vi "app - view -- guided sweep - V2.vi"() -> ()   [LabVIEW 2015]
uses:
  type - has been touched.ctl
  ctl -- name dispatcher -- action.ctl
  next chunk read-write PID -- action.ctl
  cursor action.ctl
  ctl -- name dispatcher.vi
  file -- 9w path.vi
  array -- find index - real.vi
  array -- interpolate -- i.vi
  tale of three indices.vi
  linear interpolation - real.vi
  line -- complex.vi
  Q -- check range -- i -- integer.vi
  Q -- check range -- i -- real.vi
  command stack.vi
  tale of three indices -- check state.vi
  Q - not nan -- integer.vi
  Q - not nan -- real.vi
  <vilib>/Utility/libraryn.llb/Check if File or Folder Exists.vi
  file -- read list of lines.vi
  parse -- find first line.vi
  parse -- get list of matches -- numbers.vi
  <vilib>/Utility/file.llb/Write To Spreadsheet File.vi
  <vilib>/Utility/file.llb/Write To Spreadsheet File (string).vi
  <vilib>/gmath/function.llb/Binomial Coefficient.vi
panel:
  in  "Tab Control 2":enum32{"main", "other"}(tab)
  out "Plot: Temp vs Time":cluster{dbl[], dbl[]}[](graph)=[{[0.0, 644.73684, 3070.17544, 4635.96491, 6278.50877], [60.0, 115.47619, 164.28571, 228.57143, 294.04762]}, {array[1000 elements], array[1000 elements]}]
  in  "sweep folder path":path=path "D:/Technique/RUS/LSCO/LSCO22_130814c_polished_Fenix/0_test"
  out "Plot: T slope":cluster{dbl[], dbl[]}[](graph)
  out "Plot:  dT  vs T":cluster{dbl[], dbl[]}[](graph)
  in  "divide T by":i32=1
  in  "time min":dbl(slide)=0.01167520658858774 min=-506096563.00000006 max=2129711151.0 step=0.010000000000000002 scale=0.01..1000.0 scale format="%#3_3f"
  in  "Time max":dbl(slide)=6895.4882445737985 min=-506096563.00000006 max=2129711151.0 step=0.010000000000000002 scale=0.01..10000.0 scale format="%#3_3f"
  in  "N":i32(slide)=438 min=-506096563 max=2129711151 step=1 scale=0.01..1000.0
  out "Plot: voltage":cluster{dbl[], dbl[]}[](graph)=[{[5.0, 30.0, 60.0, 100.0, 300.0], [0.1, 0.3, 0.5, 0.5, 1.5]}, {array[1000 elements], array[1000 elements]}]
  out "Plot: K/sweep vs T":cluster{dbl[], dbl[]}[](graph)
  out "Plot: (min)/sweep vs T":cluster{dbl[], dbl[]}[](graph)
  in  "Current time":timestamp=timestamp(3536522640.967544 s since 1904-01-01) format="%<%A, %b%d , %I:%M:%S%p>T"
  out "time at yellow cursor":timestamp=timestamp(3536726193.599123 s since 1904-01-01) format="%<%A, %b%d , %I:%M:%S%p>T"
  out "temperature":dbl
  in  "update bezier!":bool
  in  "update file on disk":bool
  in  "Tab Control":enum32{"fancy", "old"}(tab)
  out "new time":dbl[](array[numeric])=[0.0, 660.0877192982456, 3070.17544, 4635.96491, 6278.50877]
  out "new temperature":dbl[](array[numeric])=[60.0, 115.47619047619048, 164.28571, 228.57143, 294.04762]
  out "time":dbl[](array[numeric])=[0.0, 644.73684, 3070.17544, 4635.96491, 6278.50877]
  out "temperature":dbl[](array[numeric])=[60.0, 115.47619, 164.28571, 228.57143, 294.04762]
  in  "weights":dbl[](array[numeric])=[2.0, 5.0, 1.0, 1.0, 1.0]
  in  "weights changed":T1
  out "header":string[](array[string])=["# set temperature PID", "# Time ", "# set temperature", "# weight", "", "#cooling"]
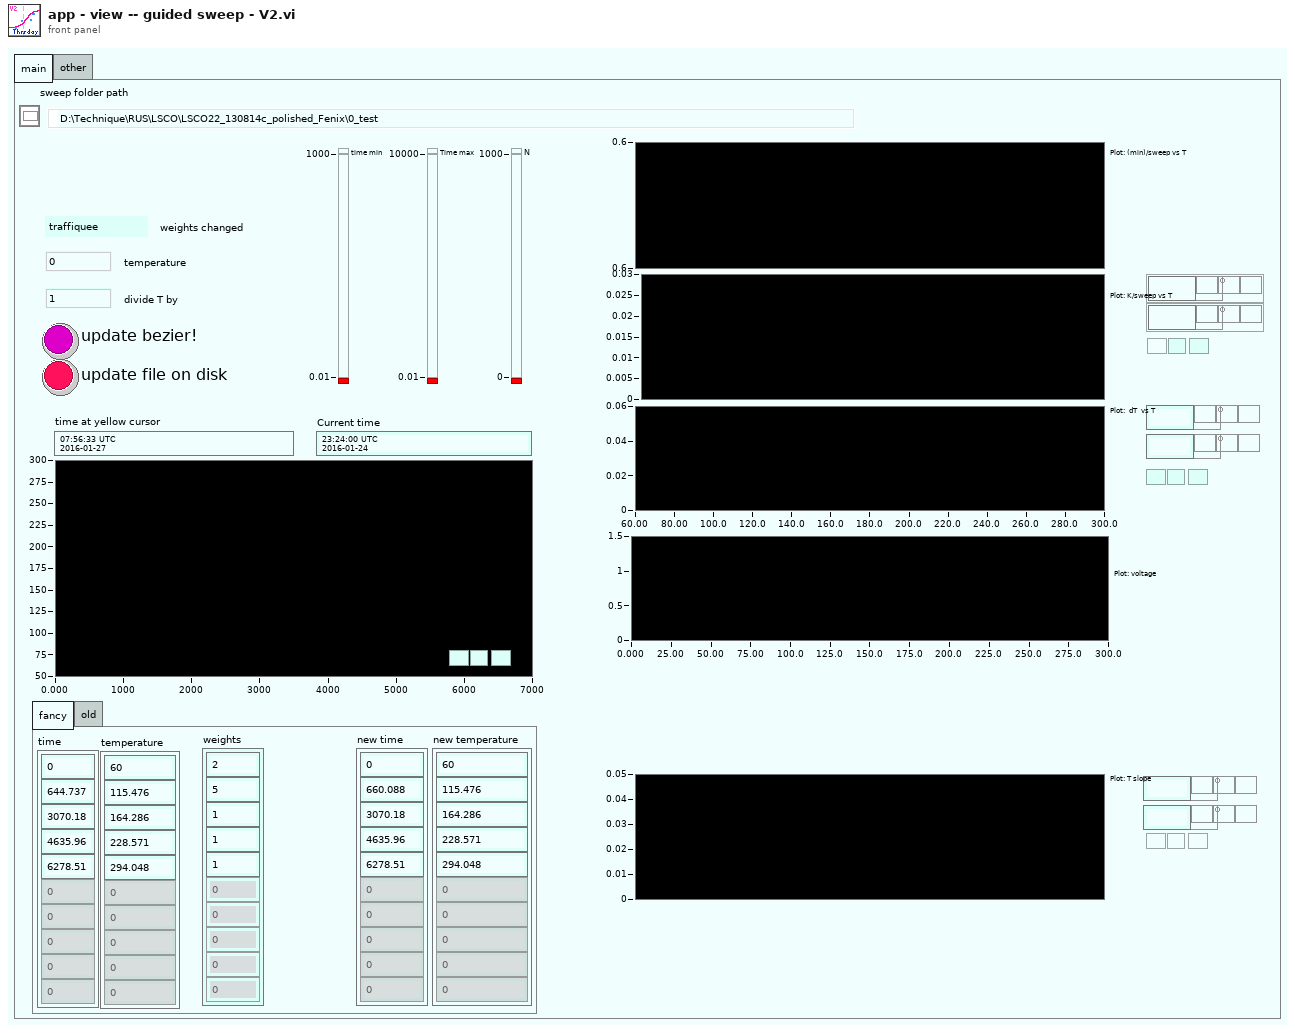
[diagram p1: front panel]
types:
  T1 = typedef "type - has been touched.ctl" = enum16{"traffiquee", "clean"}
  T2 = typedef "next chunk read-write PID -- action.ctl" = enum16{"read", "interpolate", "append col", "write", "write PID col", "append PID col", "interpolate - bezier"}
  T3 = typedef "ctl -- name dispatcher -- action.ctl" = enum16{"peak frequency", "peak frequency DUMP", "peak gamma DUMP", "peak gamma", "peak frequency TEST", "peak gamma TEST", "ultrasonic power", "time in gamma", "set temperature ", "set temperature timer", "peak default gamma", "last scan file", "peak freq gamma TEST", "peak NAMES", "errors", "P_I_D", "P", "I", "D", "power vs time", "power vs time TIMER", "void", "power log", "set temperature - SINE", "itc ltc log", "peak - time in gamma"}
  T4 = enum16{"normal", "alert", "fuzzy", "interesting", "boring", "colored"}
  T5 = typedef "cursor action.ctl" = enum16{"range", "read", "write", "check", "zoom out", "smart zoom out"}
  T6 = cluster{"temperatures":dbl[], "frequencies":dbl[]}
  T7 = cluster{"temperatures":dbl[], "frequencies":dbl[]}[]
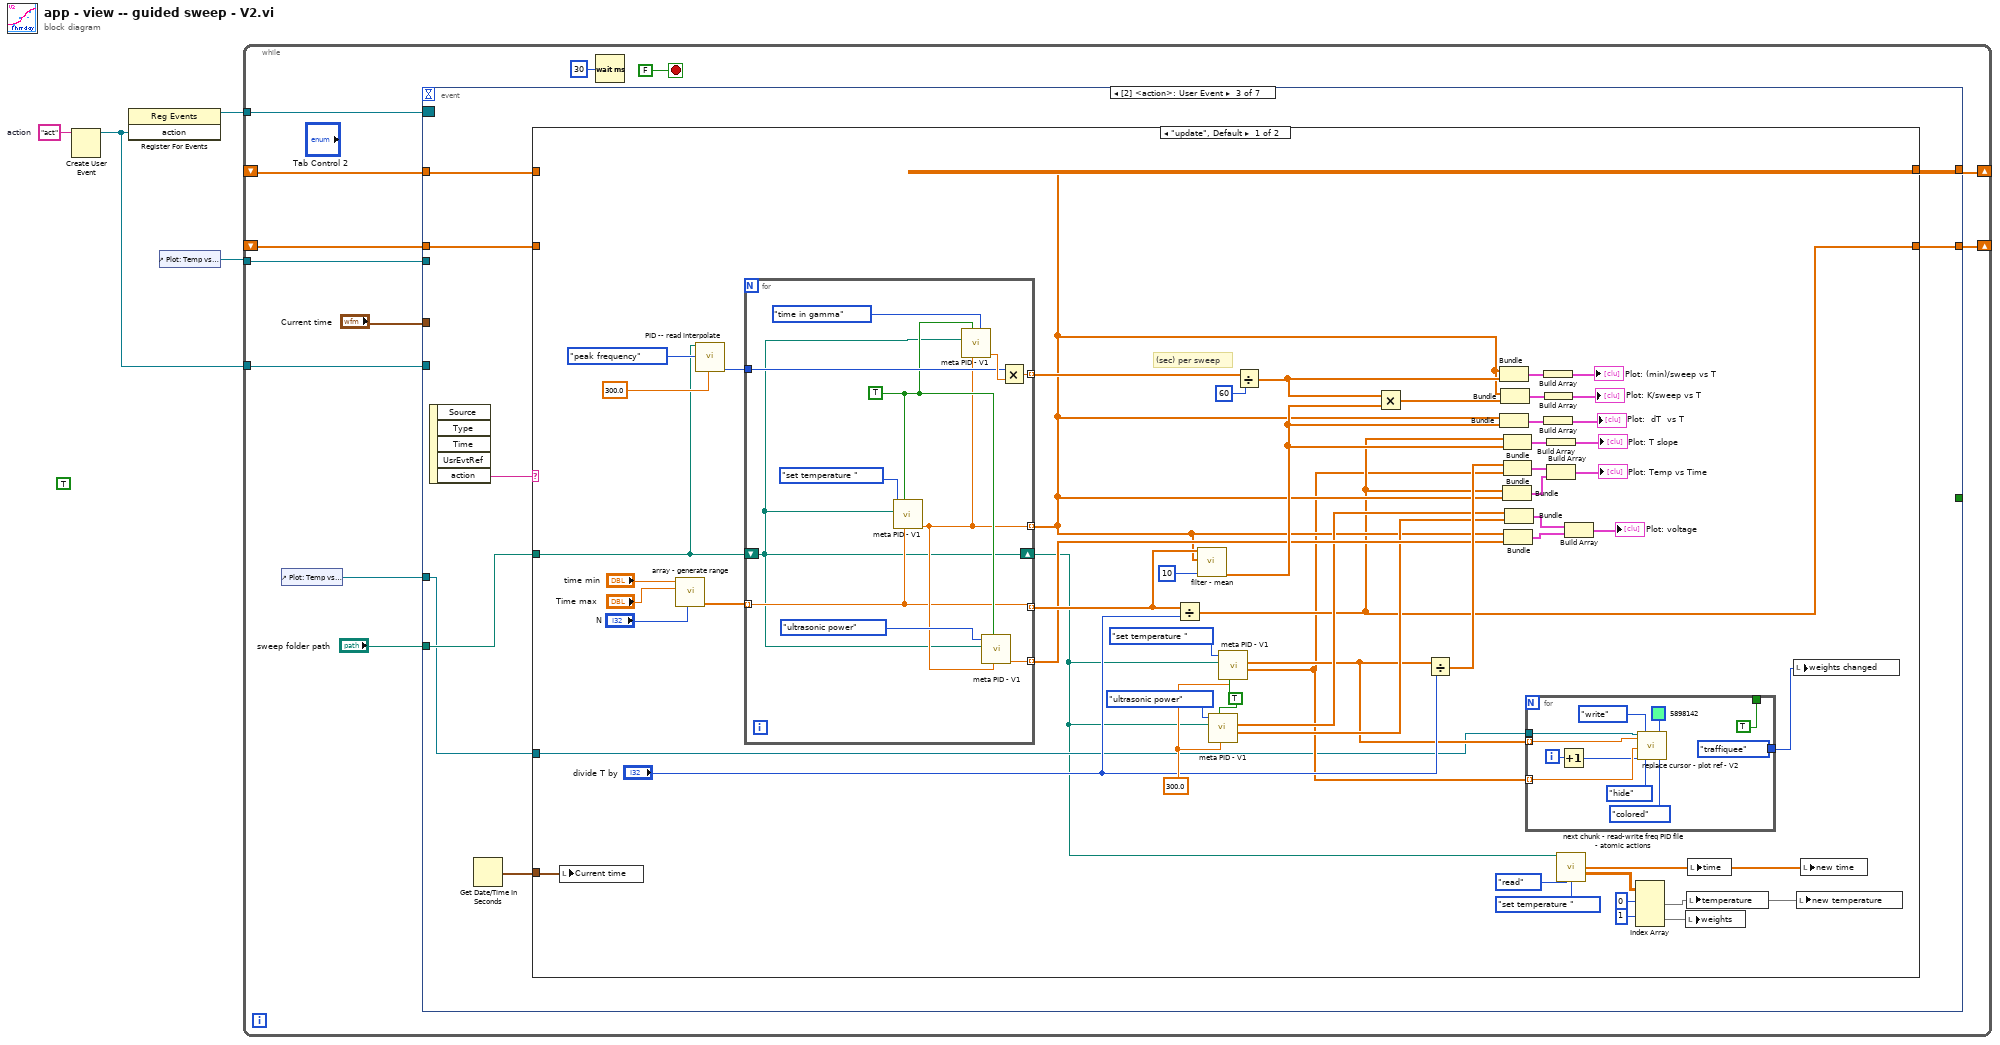
[diagram p0: block diagram]
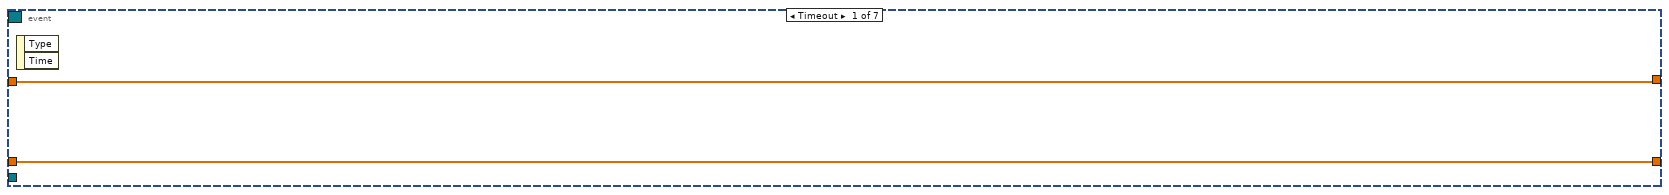
[diagram p2: hidden frame]
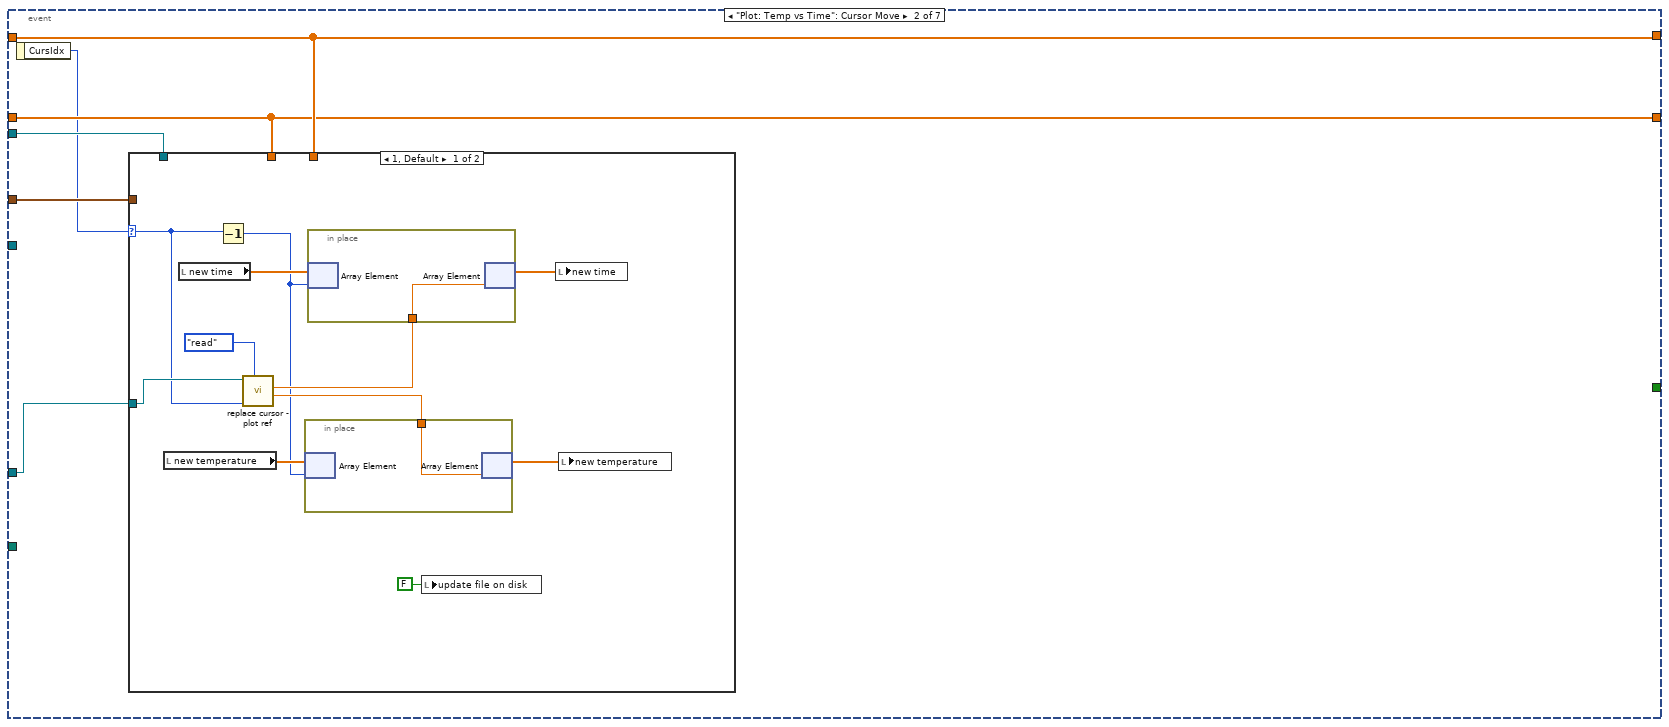
[diagram p3: hidden frame]
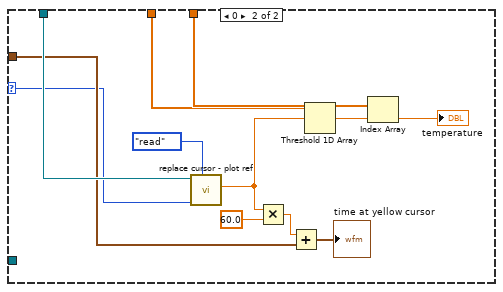
[diagram p4: hidden frame]
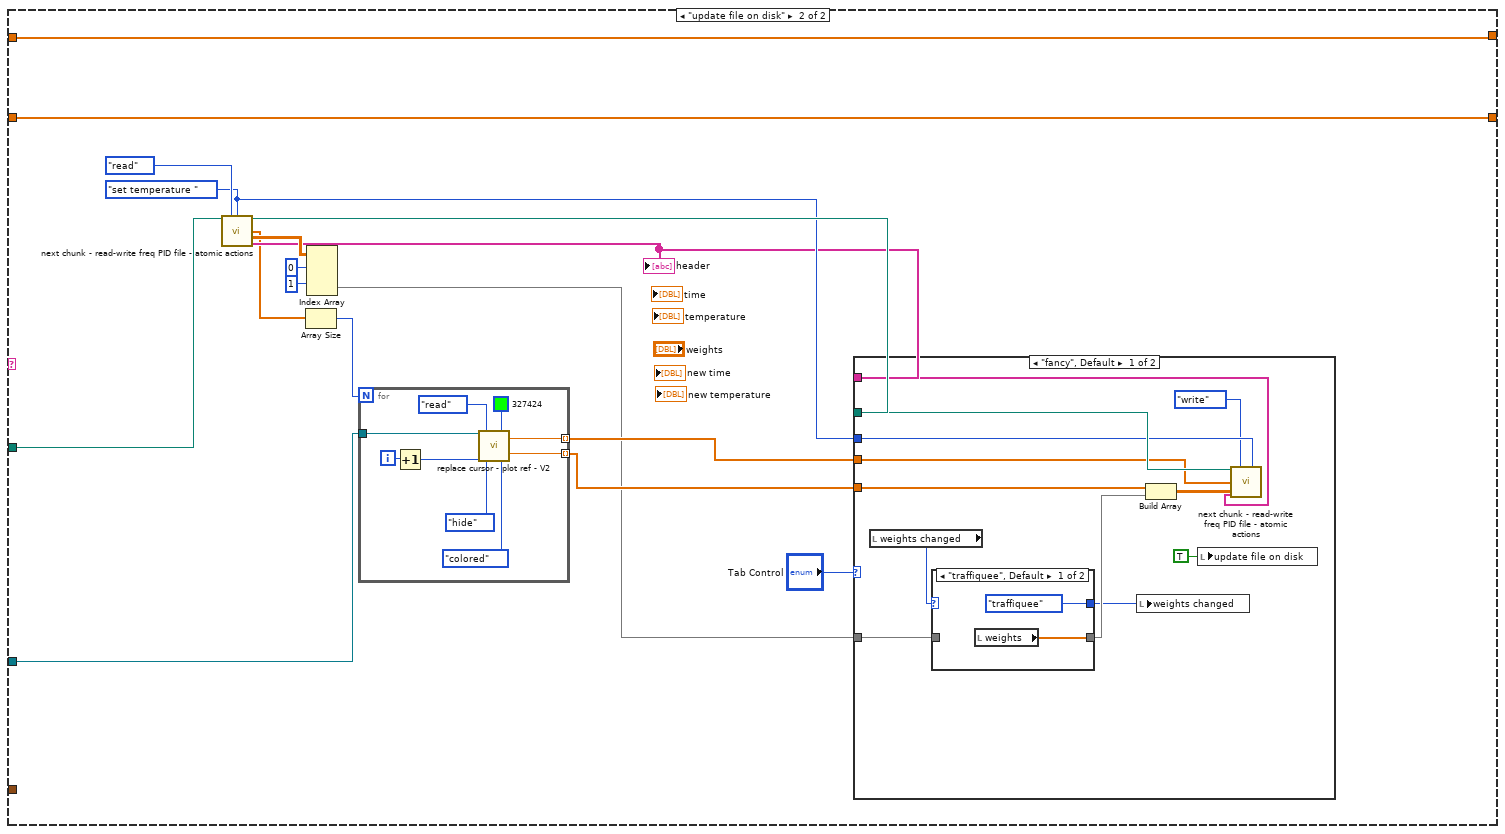
[diagram p5: hidden frame]
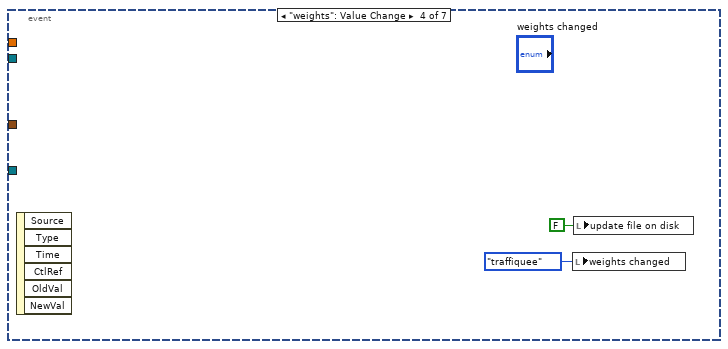
[diagram p8: hidden frame]
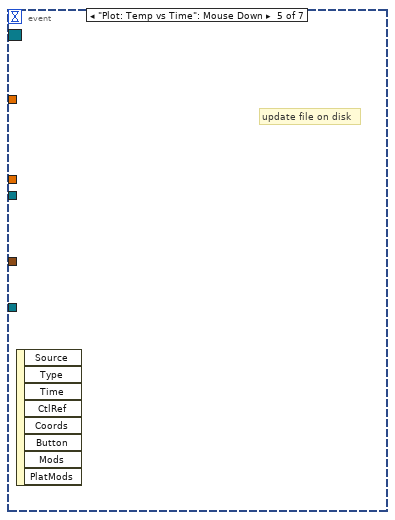
[diagram p9: hidden frame]
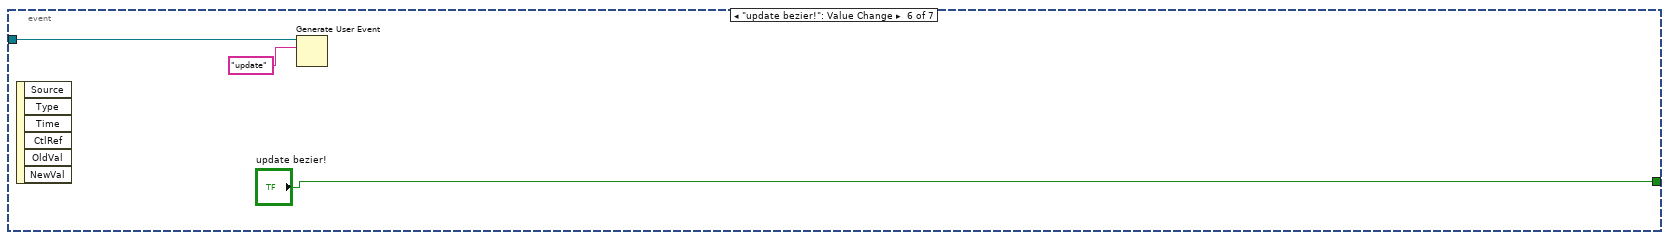
[diagram p10: hidden frame]
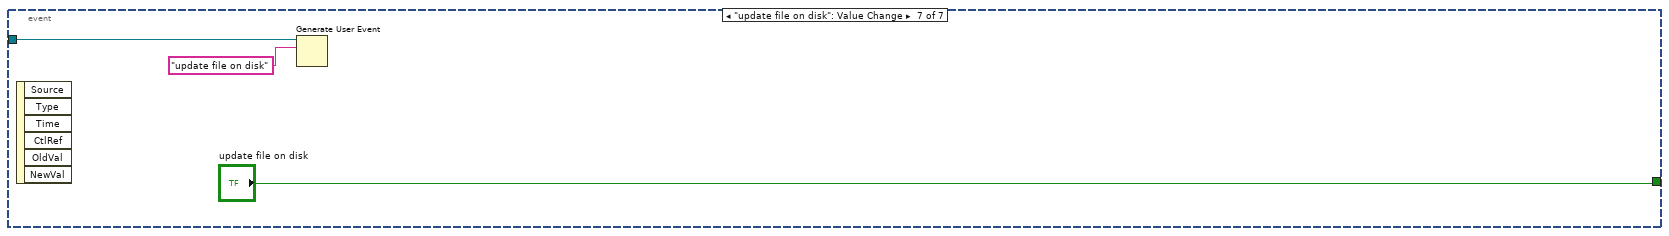
[diagram p11: hidden frame]
diagram:
  (unwired) TRUE
  w3 = "act"  # action
  n1 = Create User Event(user event datatype=w3) -> (user event=w1:refnum<user-event>)  [unwired: 1 in, 1 out]
  n2 = register-events(w1) -> (reference out=w4:refnum<event-registration>)  [unwired: 2 in, 1 out]
  n3 = control-ref of="Plot: Temp vs Time"() -> (w2:refnum<vi>)
  n4 = while {
    tunnel: w4 -> [w16]
    tunnel: w2 -> [w15]
    shift-right: [w10] -> _
    shift-left: _ -> [w12]
    shift-right: [w9] -> _
    shift-left: _ -> [w11]
    tunnel: w1 -> [w7]
    stop <- FALSE stop-if-true
    n5 = control-ref of="Plot: Temp vs Time"() -> (w6:refnum<vi>)
    n6 = event shown="[2] <action>: User Event" {
      selector: w16 -> [_ _ _ _ _ _ _]
      dyn-events: _ -> [_ _ _ _ _ _ _]
      timeout: _ -> [_ _ _ _ _ _ _]
      tunnel: w15 -> [_ w24 _ _ _ _ _]
      tunnel: "Current time" -> [_ w23 _ _ _ _ _]
      tunnel: w12 -> [w18 w22 w52 _ _ _ _]
      tunnel: w11 -> [w17 w21 w51 _ _ _ _]
      tunnel: [w18 w22 w56 _ _ _ _] -> w10
      tunnel: [w17 w21 w55 _ _ _ _] -> w9
      tunnel: w7 -> [_ _ _ _ _ w180 w183]
      tunnel: w6 -> [_ w19 w53 _ _ _ _]
      tunnel: "sweep folder path" -> [_ _ w54 _ _ _ _]
      tunnel: [_ _ _ _ _ "update bezier!" "update file on disk"] -> _
      event Timeout {
        n7 = event-data() -> ()  [unwired: 1 in, 2 out]
      }
      event "Plot: Temp vs Time": Cursor Move {
        n8 = event-data() -> ("CursIdx"=w20:i32)  [unwired: 1 in]
        n9 = case shown="1, Default" w20 {
          selector: w20 -> [w32 w38]
          tunnel: w24 -> [_ w49]
          tunnel: w23 -> [_ w45]
          tunnel: w22 -> [_ w40]
          tunnel: w21 -> [_ w39]
          tunnel: w19 -> [w33 _]
          frame 1, Default {
            n10 = local read "new temperature"() -> (w29:dbl[])
            n11 = local read "new time"() -> (w35:dbl[])
            n12 = Decrement(x=w32) -> (x-1=w26:i32)
            n13 = call "replace cursor - plot ref.vi"("action"=enum16{"", "read", "write"}."read", "cursor index"=w32, "Plot ref in"=w33) -> ("read Y"=w27:dbl, "read X"=w31:dbl)  [unwired: 6 in, 1 out]
            n14 = in-place {
              in-place-border: w27 -> [w36]
              n15 = in-place-array #1(w29, w26) -> ()  [unwired: 1 out]
              n16 = in-place-array #1(w36) -> (w28:dbl[])  [unwired: 1 out]
            }
            n17 = in-place {
              in-place-border: w31 -> [w37]
              n18 = in-place-array #2(w35, w26) -> ()  [unwired: 1 out]
              n19 = in-place-array #2(w37) -> (w30:dbl[])  [unwired: 1 out]
            }
            n20 = local write "update file on disk"(FALSE ("update file on disk")) -> ()
            n21 = local write "new time"(w30) -> ()
            n22 = local write "new temperature"(w28) -> ()
          }
          frame 0 {
            n23 = call "replace cursor - plot ref.vi"("action"=enum16{"", "read", "write"}."read", "cursor index"=w38, "Plot ref in"=w49) -> ("read X"=w43:dbl)  [unwired: 6 in, 2 out]
            n24 = Multiply(x=w43, y=60.0) -> (x*y=w46:dbl)
            n25 = Add(x=w46, y=w45) -> (x+y=→"time at yellow cursor":timestamp)
            n26 = Threshold 1D Array(2:w43, 3:w39) -> (0:w42:dbl)  [unwired: 1 in]
            n27 = Index Array(array=w40, index=w42) -> (element=→"temperature":dbl)
          }
        }
      }
      event User Event {
        n28 = event-data() -> ("action"=w57:string)  [unwired: 1 in, 4 out]
        n29 = Get Date/Time In Seconds() -> (seconds since 1Jan1904=w50:timestamp)
        n30 = case shown="\"update\", Default" w57 {
          tunnel: [w74 w148] -> w56
          tunnel: [w73 w147] -> w55
          tunnel: w54 -> [w72 w146]
          tunnel: w53 -> [w69 w150]
          tunnel: w52 -> [_ w148]
          tunnel: w51 -> [_ w147]
          tunnel: w50 -> [w58 _]
          frame "update", Default {
            w105 = TRUE ("control power PID?")
            w92 = 300.0 ("nonzero temperature")
            # "(sec) per sweep"
            n31 = local write "Current time"(w58) -> ()
            n32 = call "array - generate range.vi"("N"="N", "freq max"="Time max", "freq min"="time min") -> ("Array"=w81:dbl[])  [unwired: 7 in, 1 out]
            n33 = call "PID -- read interpolate.vi"("sweep folder path"=w72, "ctl PID file IN"=ctl_--_name_dispatcher_--_action."peak frequency", "temperature"=300.0) -> ("length out"=w90:i32)  [unwired: 11 in, 5 out]
            n34 = for {
              tunnel: w81 -> [w124] mode=indexing
              tunnel: [w128] -> w74 mode=indexing
              tunnel: w90 -> [w131]
              tunnel: [w127] -> w98 mode=indexing
              tunnel: [w126] -> w101 mode=indexing
              tunnel: [w124] -> w111 mode=indexing
              shift-right: [w123] -> w63
              shift-left: w72 -> [w123]
              w129 = TRUE ("control power PID?")
              n35 = call "meta PID - V1.vi"("input parameter"=w124, "control?"=w129, "sweep folder path"=w123, "ctl name dispatch"=ctl_--_name_dispatcher_--_action."set temperature ") -> ("bezier output"=w128:dbl)  [unwired: 4 in, 3 out]
              n36 = call "meta PID - V1.vi"("input parameter"=w128, "control?"=w129, "sweep folder path"=w123, "ctl name dispatch"=ctl_--_name_dispatcher_--_action."time in gamma") -> ("bezier output"=w132:dbl)  [unwired: 4 in, 3 out]
              n37 = call "meta PID - V1.vi"("input parameter"=w128, "control?"=w129, "sweep folder path"=w123, "ctl name dispatch"=ctl_--_name_dispatcher_--_action."ultrasonic power") -> ("bezier output"=w127:dbl)  [unwired: 4 in, 3 out]
              n38 = Multiply(x=w131, y=w132) -> (x*y=w126:dbl)
            }
            n39 = Divide(x=w111, y="divide T by") -> (x/y=w73:dbl[])
            n40 = call "filter - mean.vi"("omega  in"=w111, "z in"=w74, "window"=10) -> ("slope"=w103:dbl[])  [unwired: 13 in, 3 out]
            n41 = call "meta PID - V1.vi"("input parameter"=w92, "control?"=w105, "sweep folder path"=w63, "ctl name dispatch"=ctl_--_name_dispatcher_--_action."ultrasonic power") -> ("frequencies"=w97:dbl[], "temperatures"=w96:dbl[])  [unwired: 4 in, 2 out]
            n42 = call "meta PID - V1.vi"("input parameter"=w92, "control?"=w105, "sweep folder path"=w63, "ctl name dispatch"=ctl_--_name_dispatcher_--_action."set temperature ") -> ("frequencies"=w70:dbl[], "temperatures"=w71:dbl[])  [unwired: 4 in, 2 out]
            n43 = Divide(x=w101, y=60) -> (x/y=w108:dbl[])
            n44 = Multiply(x=w108, y=w103) -> (x*y=w104:dbl[])
            n45 = Divide(x=w71, y="divide T by") -> (x/y=w109:dbl[])
            n46 = Bundle(w74, w108) -> (w106:cluster{dbl[], dbl[]})  [unwired: 1 in]
            n47 = Bundle(w74, "slope"=w103) -> (w82:cluster{dbl[], "slope":dbl[]})  [unwired: 1 in]
            n48 = Bundle(w74, w104) -> (w99:cluster{dbl[], dbl[]})  [unwired: 1 in]
            n49 = Bundle(w73, w74) -> (w76:cluster{dbl[], dbl[]})  [unwired: 1 in]
            n50 = Bundle(w73, "slope"=w103) -> (w78:cluster{dbl[], "slope":dbl[]})  [unwired: 1 in]
            n51 = Bundle(w109, "frequencies"=w70) -> (w75:cluster{dbl[], "frequencies":dbl[]})  [unwired: 1 in]
            n52 = Bundle(w74, w98) -> (w94:cluster{dbl[], dbl[]})  [unwired: 1 in]
            n53 = Bundle("temperatures"=w96, "frequencies"=w97) -> (w93:T6)  [unwired: 1 in]
            n54 = for {
              tunnel: w71 -> [w122] mode=indexing
              tunnel: w70 -> [w121] mode=indexing
              tunnel: w69 -> [w118]
              tunnel: [TRUE ("update file on disk")] -> _
              tunnel: [type_-_has_been_touched."traffiquee" ("weights changed")] -> w59
              i -> [w120]
              n55 = Increment(x=w120) -> (x+1=w119:i32)
              n56 = call "replace cursor - plot ref - V2.vi"("Plot ref in"=w118, "new X"=w122, "new  Y"=w121, "cursor index"=w119, "cursor action"=cursor_action."write", "label"=enum16{"hide", "show x", "show y", "show (x,y)"}."hide", "Color Box"=u32 5898142, "cursor state"=T4."colored") -> ()  [unwired: 9 in, 3 out]
            }
            n57 = Build Array(w106) -> (→"Plot: (min)/sweep vs T":cluster{dbl[], dbl[]}[])
            n58 = Build Array(w82) -> (→"Plot:  dT  vs T":cluster{dbl[], "slope":dbl[]}[])
            n59 = Build Array(w99) -> (→"Plot: K/sweep vs T":cluster{dbl[], dbl[]}[])
            n60 = Build Array(w78) -> (→"Plot: T slope":cluster{dbl[], "slope":dbl[]}[])
            n61 = Build Array(w75, w76) -> (→"Plot: Temp vs Time":cluster{dbl[], "frequencies":dbl[]}[])
            n62 = call "next chunk - read-write freq PID file - atomic actions .vi"("sweep folder path"=w63, "PID action"=next_chunk_read-write_PID_--_action."read", "ctl kind IN"=ctl_--_name_dispatcher_--_action."set temperature ") -> ("temperatures"=w61:dbl[], "frequencies"=w64:dbl[][])  [unwired: 8 in, 3 out]
            n63 = Build Array(w93, w94) -> (→"Plot: voltage":T7)
            n64 = Index Array(array=w64, index (row) #1=0 ("index (row)"), index (row) #2=1 ("index (row)")) -> (element #1=w60:dbl[], element #2=w62:dbl[])  [unwired: 2 in]
            n65 = local write "weights"(w62) -> ()
            n66 = local write "temperature"(w60) -> ()
            n67 = local write "time"(w61) -> ()
            n68 = local write "weights changed"(w59) -> ()
            n69 = local write "new temperature"(w60) -> ()
            n70 = local write "new time"(w61) -> ()
          }
          frame "update file on disk" {
            w143 = ctl_--_name_dispatcher_--_action."set temperature " ("ctl kind IN")
            n71 = call "next chunk - read-write freq PID file - atomic actions .vi"("sweep folder path"=w146, "PID action"=next_chunk_read-write_PID_--_action."read", "ctl kind IN"=w143) -> ("sweep folder path out"=w144:path, "temperatures"=w138:dbl[], "frequencies"=w140:dbl[][], "header"=w139:string[])  [unwired: 8 in, 1 out]
            "header" <- w139
            n72 = Array Size(array=w138) -> (size(s)=w149:i32)
            n73 = Index Array(array=w140, index (row) #1=0 ("index (row)"), index (row) #2=1 ("index (row)")) -> (element #2=w134:dbl[])  [unwired: 2 in, 1 out]
            n74 = for {
              N: w149 -> [_]
              tunnel: w150 -> [w173]
              tunnel: [w168] -> w137 mode=indexing
              tunnel: [w167] -> w135 mode=indexing
              i -> [w175]
              n75 = Increment(x=w175) -> (x+1=w174:i32)
              n76 = call "replace cursor - plot ref - V2.vi"("Plot ref in"=w173, "cursor index"=w174, "cursor action"=cursor_action."read", "label"=enum16{"hide", "show x", "show y", "show (x,y)"}."hide", "Color Box"=u32 327424, "cursor state"=T4."colored") -> ("read X"=w168:dbl, "read Y"=w167:dbl)  [unwired: 11 in, 1 out]
            }
            n77 = case shown="\"fancy\", Default" "Tab Control" {
              tunnel: w144 -> [w162 _]
              tunnel: w143 -> [w161 _]
              tunnel: w139 -> [w159 _]
              tunnel: w137 -> [w158 _]
              tunnel: w135 -> [w156 _]
              tunnel: w134 -> [w153 _]
              frame "fancy", Default {
                n78 = local read "weights changed"() -> (w155:T1)
                n79 = case shown="\"traffiquee\", Default" w155 {
                  selector: w155 -> [_ w165]
                  tunnel: [w164 w166] -> w154
                  tunnel: w153 -> [_ w166]
                  tunnel: [type_-_has_been_touched."traffiquee" ("weights changed") w165] -> w151
                  frame "traffiquee", Default {
                    n80 = local read "weights"() -> (w164:dbl[])
                  }
                  frame "clean" {
                  }
                }
                n81 = local write "weights changed"(w151) -> ()
                n82 = Build Array(w156, w154) -> (w152:dbl[][])
                n83 = local write "update file on disk"(TRUE ("update file on disk")) -> ()
                n84 = call "next chunk - read-write freq PID file - atomic actions .vi"("sweep folder path"=w162, "PID action"=next_chunk_read-write_PID_--_action."write", "ctl kind OUT"=w161, "temperatures IN"=w158, "frequencies IN"=w152, "header IN"=w159) -> ()  [unwired: 5 in, 5 out]
              }
              frame "old" {
              }
            }
          }
        }
      }
      event "weights": Value Change {
        n85 = event-data() -> ()  [unwired: 1 in, 6 out]
        n86 = local write "weights changed"(type_-_has_been_touched."traffiquee" ("has been touched")) -> ()
        n87 = local write "update file on disk"(FALSE ("update file on disk")) -> ()
      }
      event "Plot: Temp vs Time": Mouse Down {
        # "update file on disk"
        n88 = event-data() -> ()  [unwired: 1 in, 8 out]
      }
      event "update bezier!": Value Change {
        n89 = event-data() -> ()  [unwired: 1 in, 6 out]
        n90 = Generate User Event(user event=w180, event data cluster="update" ("event data")) -> ()  [unwired: 2 in, 2 out]
      }
      event "update file on disk": Value Change {
        n91 = event-data() -> ()  [unwired: 1 in, 6 out]
        n92 = Generate User Event(user event=w183, event data cluster="update file on disk" ("event data")) -> ()  [unwired: 2 in, 2 out]
      }
    }
    n93 = Wait (ms)(milliseconds to wait=u32 30) -> ()  [unwired: 1 out]
  }
